vi "Translate Data.vi"(8 "error in":errorcluster, 10 "DataBuffer":string, 11 "Alicat_MC in":refnum<class "Alicat_MC.lvclass">) -> (0 "error out":errorcluster, 2 "Data":refnum<class "Data.lvclass">, 3 "Alicat_MC out":refnum<class "Alicat_MC.lvclass">)   [LabVIEW 2015, in "Alicat.lvlib" / "Alicat_MC.lvclass"]
doc: "VI used to translate the data buffer to something meaningful (implementation dependent). This VI must be overridden."
uses:
  Alicat_MC.lvclass
  Reusable/Data/Data.lvclass
  Data/MC/AlicatMCData.lvclass
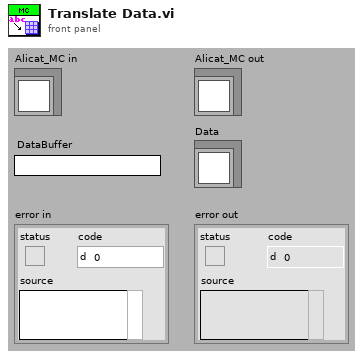
[diagram p1: front panel]
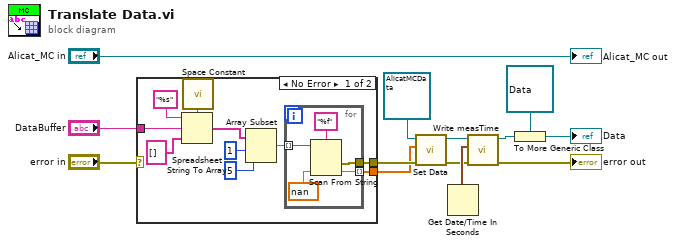
[diagram p0: block diagram]
diagram:
  n1 = case shown="No Error" "error in" {
    selector: "error in" -> [_ w29]
    tunnel: "DataBuffer" -> [w20 _]
    tunnel: [w15 _] -> w4
    tunnel: [w19 w29] -> w8
    frame No Error {
      n2 = call <vilib>:"Space Constant.vi"() -> ("String"=w22:string)
      n3 = Spreadsheet String To Array(delimiter (Tab)=w22, format string="%s", spreadsheet string=w20, array type (2D Dbl)=string[] []) -> (array=w18:string[])
      n4 = Array Subset(array=w18, index=1, length=5) -> (w16:string[])
      n5 = for {
        tunnel: w16 -> [w24] mode=indexing
        tunnel: [w26] -> w15 mode=indexing
        tunnel: [w25] -> w19
        n6 = Scan From String(format string="%f", input string=w24, default 1=sgl nan ("default value 1")) -> (error out=w25:errorcluster, output 1=w26:sgl)  [unwired: 2 in, 2 out]
      }
    }
    frame Error {
    }
  }
  n7 = call "Set Data.vi"("error in"=w8, "DataIn"=w4, "AlicatMData in"=refnum<class "AlicatMCData.lvclass"> refnum ("AlicatMCData.lvclass")) -> ("error out"=w7:errorcluster, "AlicatMData out"=w10:refnum<class "AlicatMCData.lvclass">)  [unwired: 7 in]
  n8 = Get Date/Time In Seconds() -> (seconds since 1Jan1904=w9:timestamp)
  n9 = call "Write measTime.vi"("error in (no error)"=w7, "measTime"=w9, "Data in"=w10) -> ("error out"=→"error out":errorcluster, "Data out"=w3:refnum<class "AlicatMCData.lvclass">)  [unwired: 7 in]
  n10 = To More Generic Class(target class=refnum<class "Data.lvclass"> refnum ("Data"), reference=w3) -> (generic class reference=→"Data":refnum<class "Data.lvclass">)
  "Alicat_MC out" <- "Alicat_MC in"
